vi "SetBool.vi"(8 "error in (no error)":errorcluster, 10 "Bool":bool, 11 "Animal in":refnum<class "Animal.lvclass">) -> (0 "error out":errorcluster, 3 "Animal out":refnum<class "Animal.lvclass">)   [LabVIEW 2018, in "Animal.lvclass"]
uses:
  Animal.lvclass
  Animal.lvclass/Animal.ctl
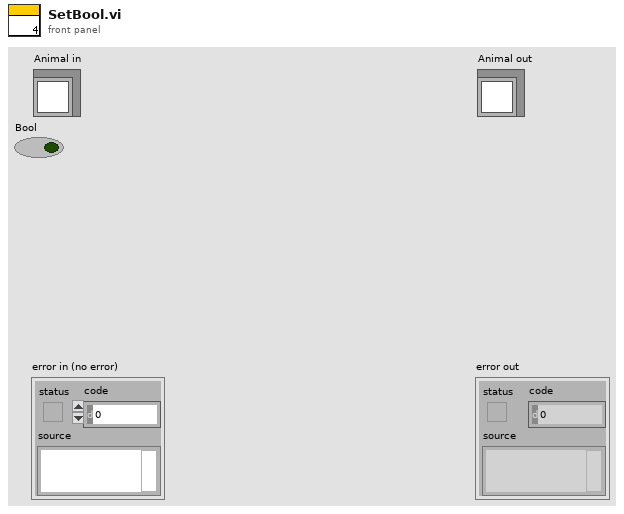
[diagram p1: front panel]
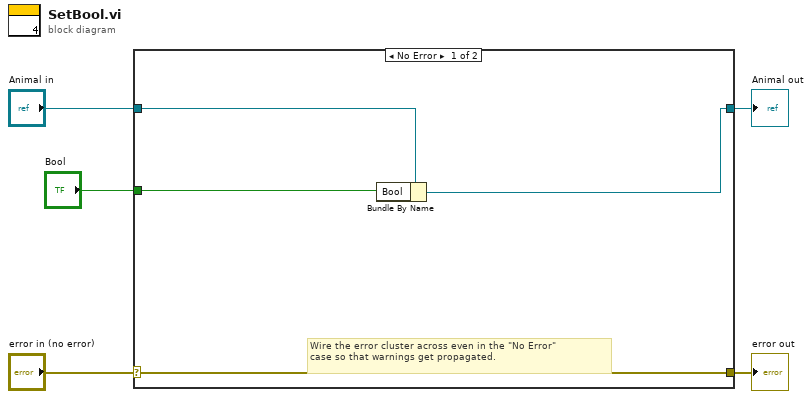
[diagram p0: block diagram]
diagram:
  n1 = case shown="No Error" "error in (no error)" {
    selector: "error in (no error)" -> [w9 w11]
    tunnel: [w9 w11] -> w4
    tunnel: [w7 w10] -> w2
    tunnel: "Animal in" -> [w8 w10]
    tunnel: "Bool" -> [w6 _]
    frame No Error {
      # "Wire the error cluster across even in the \"No Error\"\ncase so that warnings get propagated."
      n2 = Bundle By Name(cluster=w8, "Bool"=w6) -> (w7:refnum<class "Animal.lvclass">)
    }
    frame Error {
    }
  }
  "error out" <- w4
  "Animal out" <- w2
